vi "Step initialise.vi"(10 "file path (dialog if empty)":path, 11 "Step array":T1) -> (2 "all rows":string[][](array[string]), 3 "Step array out":T1)   [LabVIEW 2014]
uses:
  Controls/Step array.ctl
  Step/Control/Step name enum.ctl
  <vilib>/Utility/file.llb/Read From Spreadsheet File (string).vi
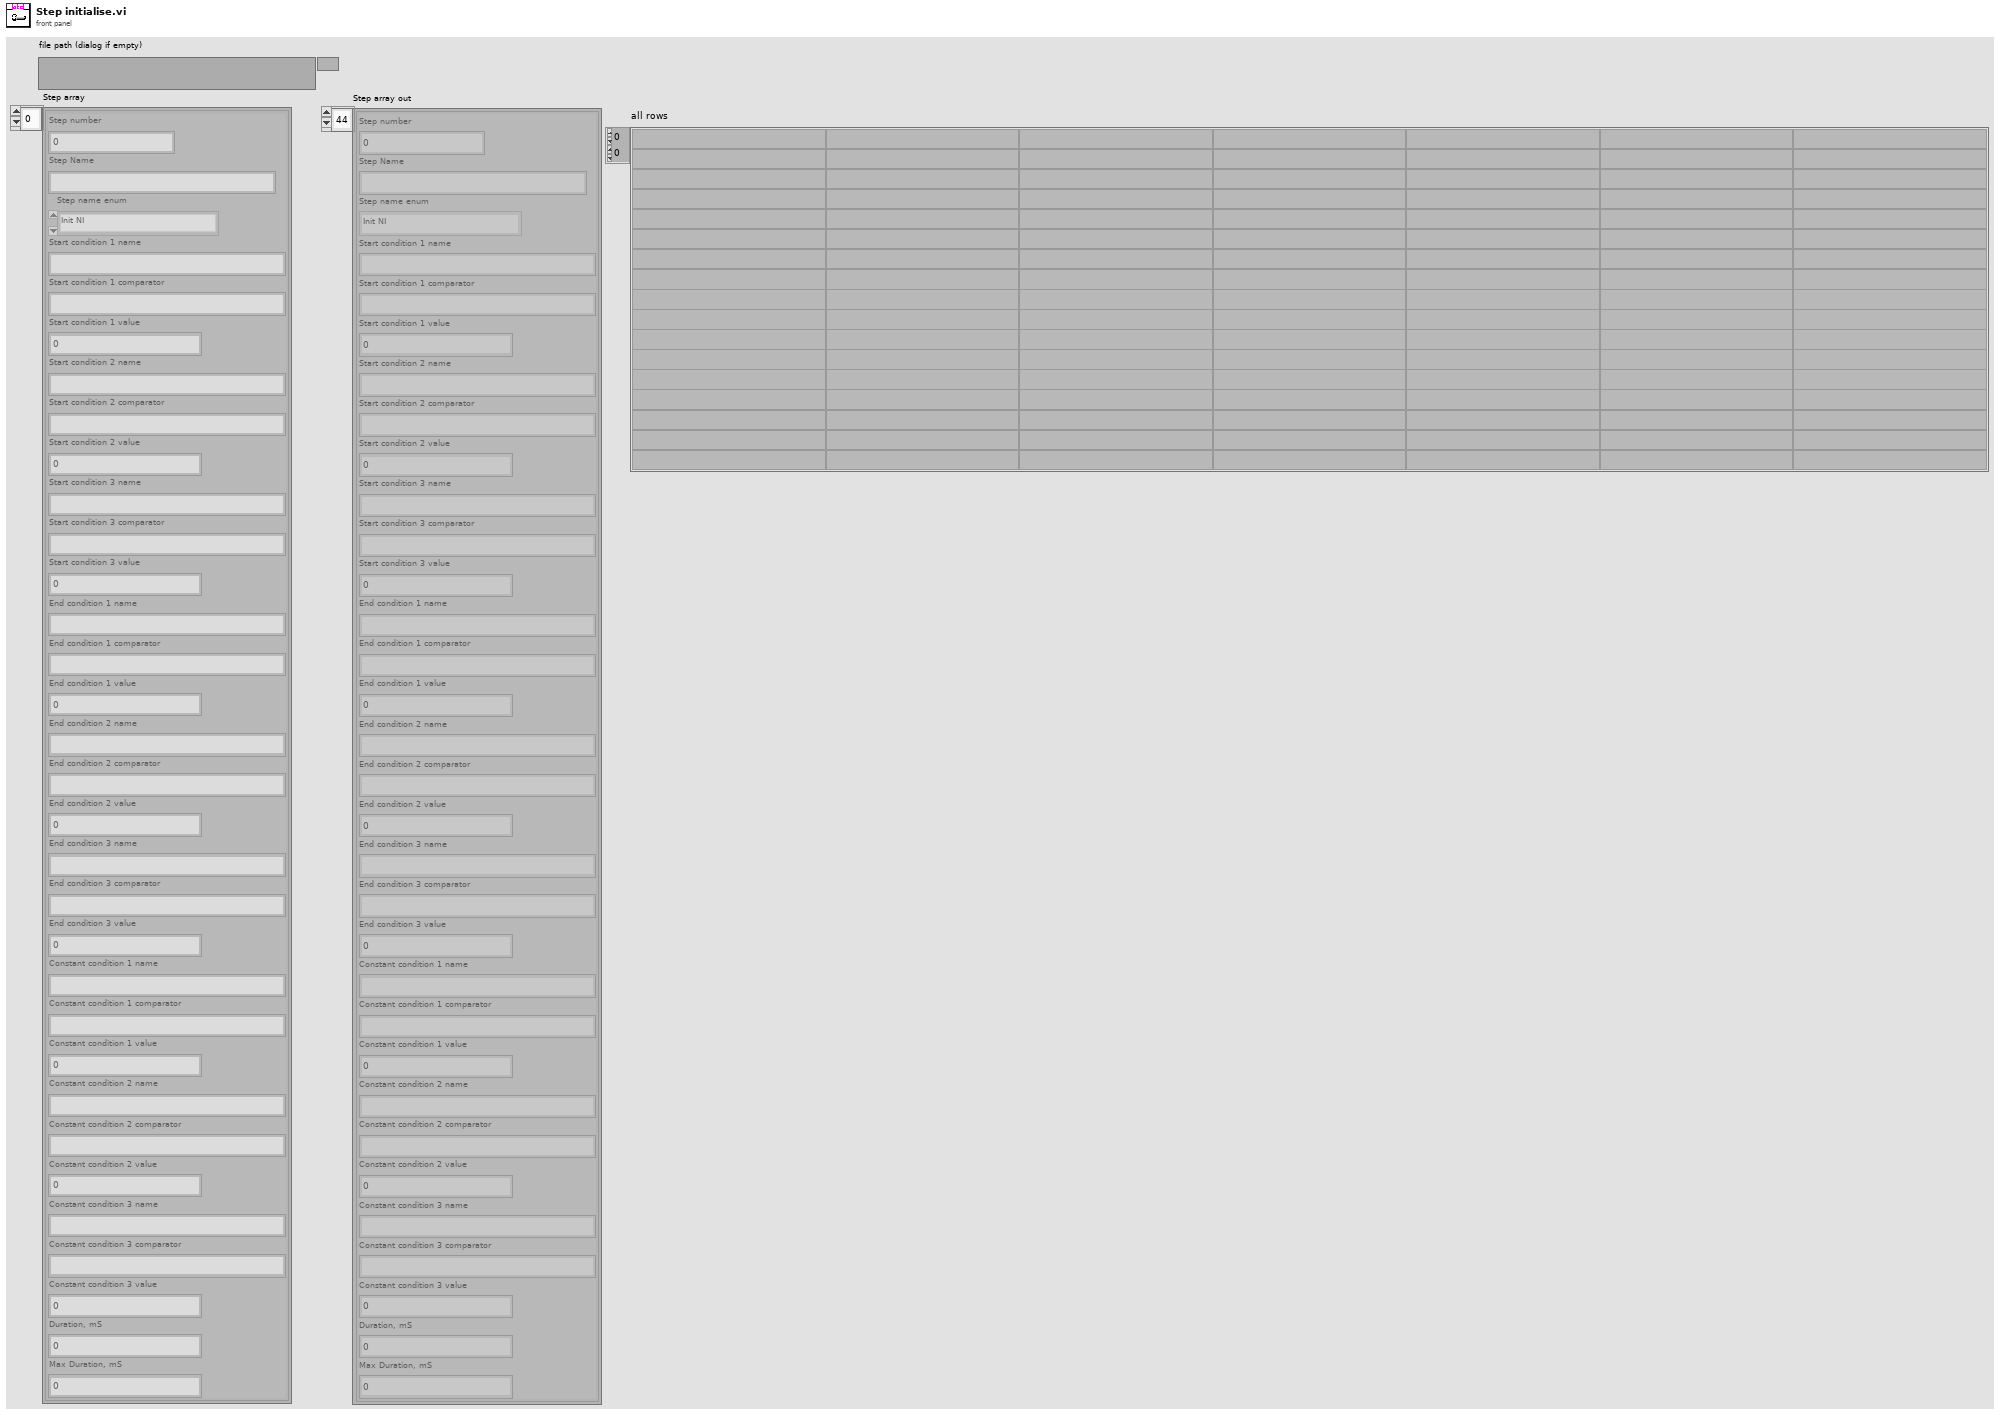
[diagram p1: front panel]
types:
  T1 = typedef "Step array.ctl" = cluster{"Step number":i32, "Step Name":string, "Step name enum":T2, "Start condition 1 name":string, "Start condition 1 comparator":string, "Start condition 1 value":dbl, "Start condition 2 name":string, "Start condition 2 comparator":string, "Start condition 2 value":dbl, "Start condition 3 name":string, "Start condition 3 comparator":string, "Start condition 3 value":dbl, "End condition 1 name":string, "End condition 1 comparator":string, "End condition 1 value":dbl, "End condition 2 name":string, "End condition 2 comparator":string, "End condition 2 value":dbl, "End condition 3 name":string, "End condition 3 comparator":string, "End condition 3 value":dbl, "Constant condition 1 name":string, "Constant condition 1 comparator":string, "Constant condition 1 value":dbl, "Constant condition 2 name":string, "Constant condition 2 comparator":string, "Constant condition 2 value":dbl, "Constant condition 3 name":string, "Constant condition 3 comparator":string, "Constant condition 3 value":dbl, "Duration, mS":dbl, "Max Duration, mS":dbl}[]
  T2 = typedef "Step name enum.ctl" = enum16{"Default", "Idle", "Init Ard", "Init SM", "Init NI", "Run", "Close"}
  T3 = cluster{"Step number":i32, "Step Name":string, "Step name enum":T2, "Start condition 1 name":string, "Start condition 1 comparator":string, "Start condition 1 value":dbl, "Start condition 2 name":string, "Start condition 2 comparator":string, "Start condition 2 value":dbl, "Start condition 3 name":string, "Start condition 3 comparator":string, "Start condition 3 value":dbl, "End condition 1 name":string, "End condition 1 comparator":string, "End condition 1 value":dbl, "End condition 2 name":string, "End condition 2 comparator":string, "End condition 2 value":dbl, "End condition 3 name":string, "End condition 3 comparator":string, "End condition 3 value":dbl, "Constant condition 1 name":string, "Constant condition 1 comparator":string, "Constant condition 1 value":dbl, "Constant condition 2 name":string, "Constant condition 2 comparator":string, "Constant condition 2 value":dbl, "Constant condition 3 name":string, "Constant condition 3 comparator":string, "Constant condition 3 value":dbl, "Duration, mS":dbl, "Max Duration, mS":dbl}
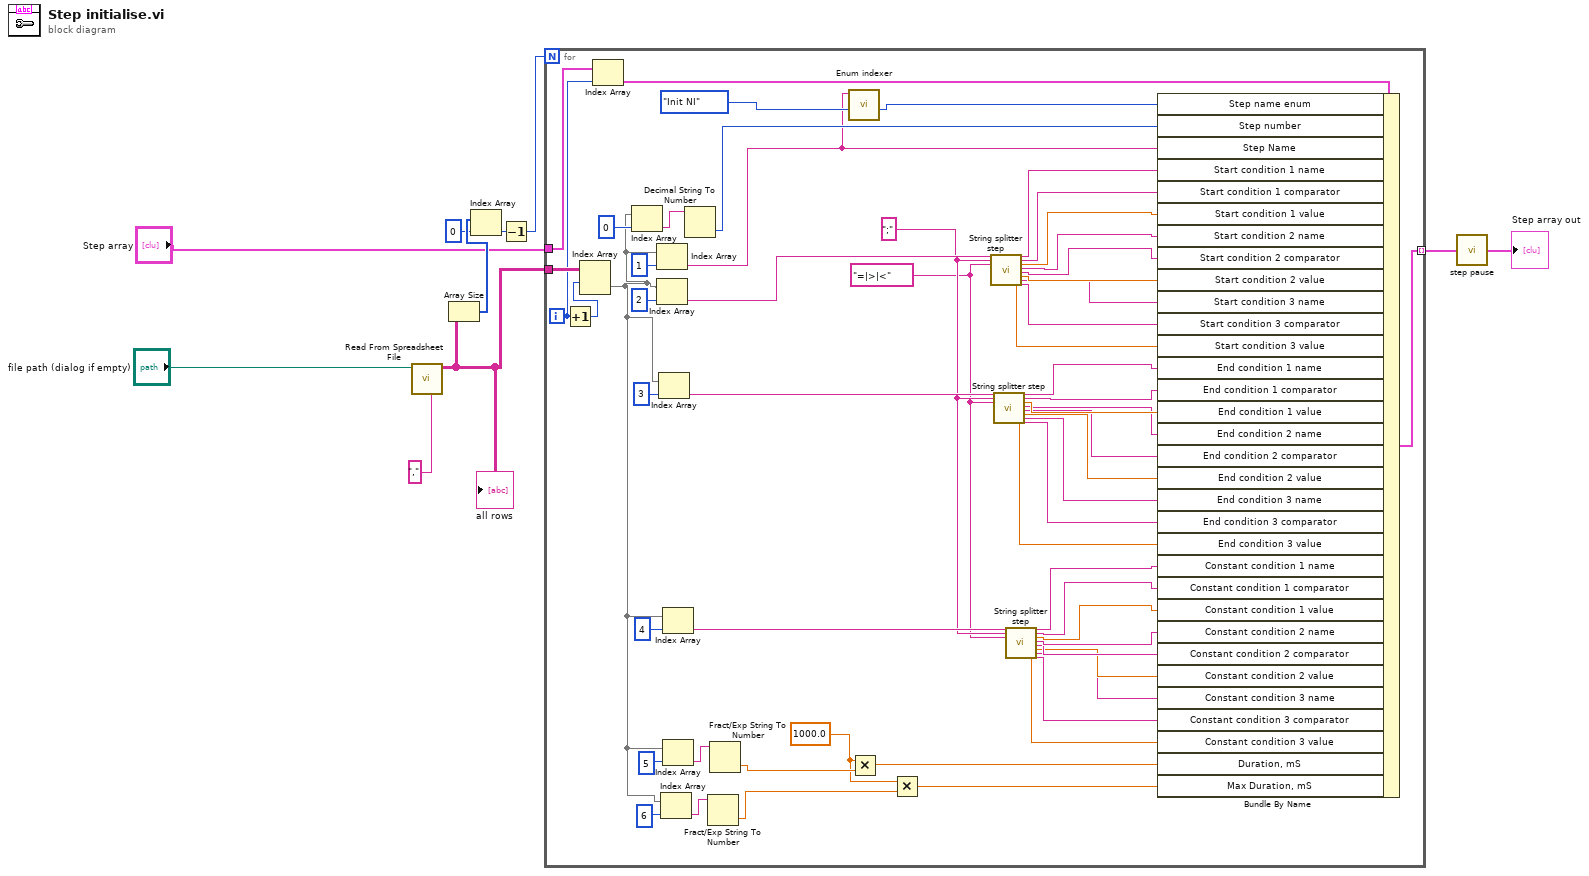
[diagram p0: block diagram]
diagram:
  n1 = call-poly <vilib>:"Read From Spreadsheet File.vi"("delimiter (\\t)"="," ("delimiter (\\t)"), "file path (dialog if empty)"="file path (dialog if empty)") -> ("all rows"=w6:string[][])  [unwired: 5 in, 4 out]
  "all rows" <- w6
  n2 = Array Size(array=w6) -> (size(s)=w10:i32[])
  n3 = Index Array(array=w10, index=0) -> (element=w7:i32)
  n4 = Decrement(x=w7) -> (x-1=w8:i32)
  n5 = for {
    N: w8 -> [_]
    tunnel: w6 -> [w68]
    tunnel: "Step array" -> [w59]
    tunnel: [w21] -> w2 mode=indexing
    i -> [w58]
    w16 = 1000.0
    w20 = "=|>|<" ("regular expression")
    w23 = ";" ("regular expression")
    n6 = Increment(x=w58) -> (x+1=w67:i32)
    n7 = Index Array(array=w68, index (row)=w67) -> (element=w26:string[])  [unwired: 1 in]
    n8 = Index Array(array=w59, index=w58) -> (element=w22:T3)
    n9 = Index Array(array=w26, index=0) -> (element=w65:string)
    n10 = Index Array(array=w26, index=1) -> (element=w12:string)
    n11 = Index Array(array=w26, index=2) -> (element=w57:string)
    n12 = Index Array(array=w26, index=3) -> (element=w47:string)
    n13 = Index Array(array=w26, index=6) -> (element=w24:string)
    n14 = Index Array(array=w26, index=4) -> (element=w37:string)
    n15 = Index Array(array=w26, index=5) -> (element=w25:string)
    n16 = Decimal String To Number(string=w65) -> (number=w19:i32)  [unwired: 2 in, 1 out]
    n17 = Fract/Exp String To Number(string=w24) -> (number=w18:dbl)  [unwired: 3 in, 1 out]
    n18 = Fract/Exp String To Number(string=w25) -> (number=w17:dbl)  [unwired: 3 in, 1 out]
    n19 = call "Enum indexer.vi"("Step name enum in"=Step_name_enum."Init NI" ("Step name enum"), "Step name"=w12) -> ("Step name enum out"=w11:T2)  [unwired: 9 in]
    n20 = Multiply(x=w16, y=w17) -> (x*y=w14:dbl)
    n21 = Multiply(x=w16, y=w18) -> (x*y=w15:dbl)
    n22 = call "String splitter step.vi"("Input string"=w57, "regular expression 1"=w23, "regular expression 2"=w20) -> ("Condition value 3"=w48:dbl, "Condition name 1"=w56:string, "Condition comparator 1"=w55:string, "Condition value 1"=w54:dbl, "Condition name 2"=w53:string, "Condition comparator 2"=w52:string, "Condition value 2"=w51:dbl, "Condition name 3"=w50:string, "Condition comparator 3"=w49:string)  [unwired: 16 in]
    n23 = call "String splitter step.vi"("Input string"=w47, "regular expression 1"=w23, "regular expression 2"=w20) -> ("Condition value 3"=w38:dbl, "Condition name 1"=w46:string, "Condition comparator 1"=w45:string, "Condition value 1"=w44:dbl, "Condition name 2"=w43:string, "Condition comparator 2"=w42:string, "Condition value 2"=w41:dbl, "Condition name 3"=w40:string, "Condition comparator 3"=w39:string)  [unwired: 16 in]
    n24 = call "String splitter step.vi"("Input string"=w37, "regular expression 1"=w23, "regular expression 2"=w20) -> ("Condition value 3"=w28:dbl, "Condition name 1"=w36:string, "Condition comparator 1"=w35:string, "Condition value 1"=w34:dbl, "Condition name 2"=w33:string, "Condition comparator 2"=w32:string, "Condition value 2"=w31:dbl, "Condition name 3"=w30:string, "Condition comparator 3"=w29:string)  [unwired: 16 in]
    n25 = Bundle By Name(cluster=w22, "Step name enum"=w11, "Step number"=w19, "Step Name"=w12, "Start condition 1 name"=w56, "Start condition 1 comparator"=w55, "Start condition 1 value"=w54, "Start condition 2 name"=w53, "Start condition 2 comparator"=w52, "Start condition 2 value"=w51, "Start condition 3 name"=w50, "Start condition 3 comparator"=w49, "Start condition 3 value"=w48, "End condition 1 name"=w46, "End condition 1 comparator"=w45, "End condition 1 value"=w44, "End condition 2 name"=w43, "End condition 2 comparator"=w42, "End condition 2 value"=w41, "End condition 3 name"=w40, "End condition 3 comparator"=w39, "End condition 3 value"=w38, "Constant condition 1 name"=w36, "Constant condition 1 comparator"=w35, "Constant condition 1 value"=w34, "Constant condition 2 name"=w33, "Constant condition 2 comparator"=w32, "Constant condition 2 value"=w31, "Constant condition 3 name"=w30, "Constant condition 3 comparator"=w29, "Constant condition 3 value"=w28, "Duration, mS"=w14, "Max Duration, mS"=w15) -> (w21:T3)
  }
  n26 = call "step pause.vi"("Step array"=w2) -> ("step array out"=→"Step array out":T1)  [unwired: 4 in]
